vi "RelativePosition_KCubeInertial.vi"(9 "decrease/reverse":bool, 10 "increase/forward":bool, 11 ".NET Refnum in":refnum<k24>) -> ()   [LabVIEW 2019]
doc: "run relative position for inertial motor (no settings)"
uses:
  D:/Victor Sun/optical trap control/Kinesis/Thorlabs.MotionControl.KCube.InertialMotorCLI.dll
  Kinesis/Thorlabs.MotionControl.KCube.InertialMotorCLI.dll
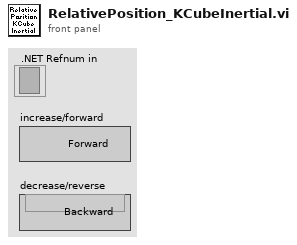
[diagram p1: front panel]
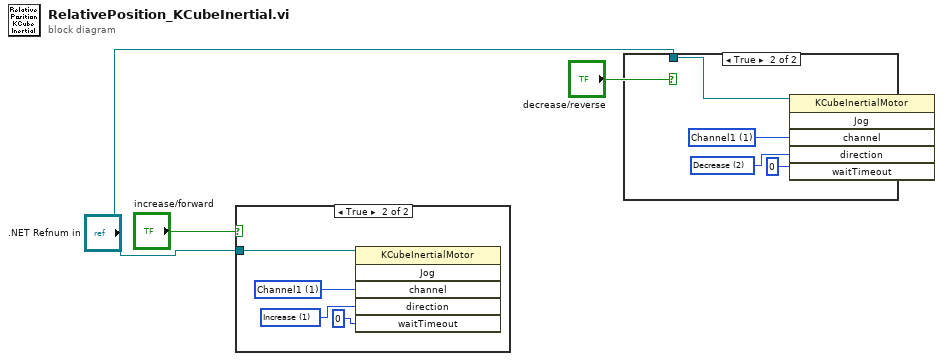
[diagram p0: block diagram]
diagram:
  n1 = case shown="True" "increase/forward" {
    tunnel: ".NET Refnum in" -> [_ w7]
    frame False {
    }
    frame True {
      w4 = 1 items=["Increase"=1, "Decrease"=2] ("direction")
      w6 = 1 items=["Channel1"=1, "Channel2"=2, "Channel3"=3, "Channel4"=4] ("channel")
      n2 = invoke class="KCubeInertialMotor" method="Jog"(reference=w7, "channel"=w6, "direction"=w4, "waitTimeout"=0) -> ()  [unwired: 2 in, 6 out]
    }
  }
  n3 = case shown="True" "decrease/reverse" {
    tunnel: ".NET Refnum in" -> [_ w11]
    frame False {
    }
    frame True {
      w8 = 2 items=["Increase"=1, "Decrease"=2] ("direction")
      w10 = 1 items=["Channel1"=1, "Channel2"=2, "Channel3"=3, "Channel4"=4] ("channel")
      n4 = invoke class="KCubeInertialMotor" method="Jog"(reference=w11, "channel"=w10, "direction"=w8, "waitTimeout"=0) -> ()  [unwired: 2 in, 6 out]
    }
  }
